vi "Global Log Handling Capability Example.vi"() -> ()   [LabVIEW 2017]
uses:
  user.lib/_NEVSTOP/Communicable State Machine(CSM)/Utility/_support/Periodic String Filter Level.ctl
  user.lib/_NEVSTOP/Communicable State Machine(CSM)/Utility/Periodic String Filter Setting.ctl
  user.lib/_NEVSTOP/Communicable State Machine(CSM)/Communicable State Machine.lvlib
  user.lib/_NEVSTOP/Communicable State Machine(CSM)/addons/Watchdog/CSM Watchdog.lvlib
  user.lib/_NEVSTOP/Communicable State Machine(CSM)/_Shared/CSM Shared.lvlib
panel:
  in  "Module Num":i32=30
  out "log handling Speed(#/s)":dbl(graph)
  out "Since Exiting(s)":dbl format="%.2f"
  out "LogInQ":i32
  out "State History":string
  out "log handling Speed(#/s)":dbl
  out "LogInQ changing Speed(#/s)":dbl
  out "Level":T1
  out "Module Names":string[](array[string])
  in  "Exit Modules":bool
  # "Set before run VI"
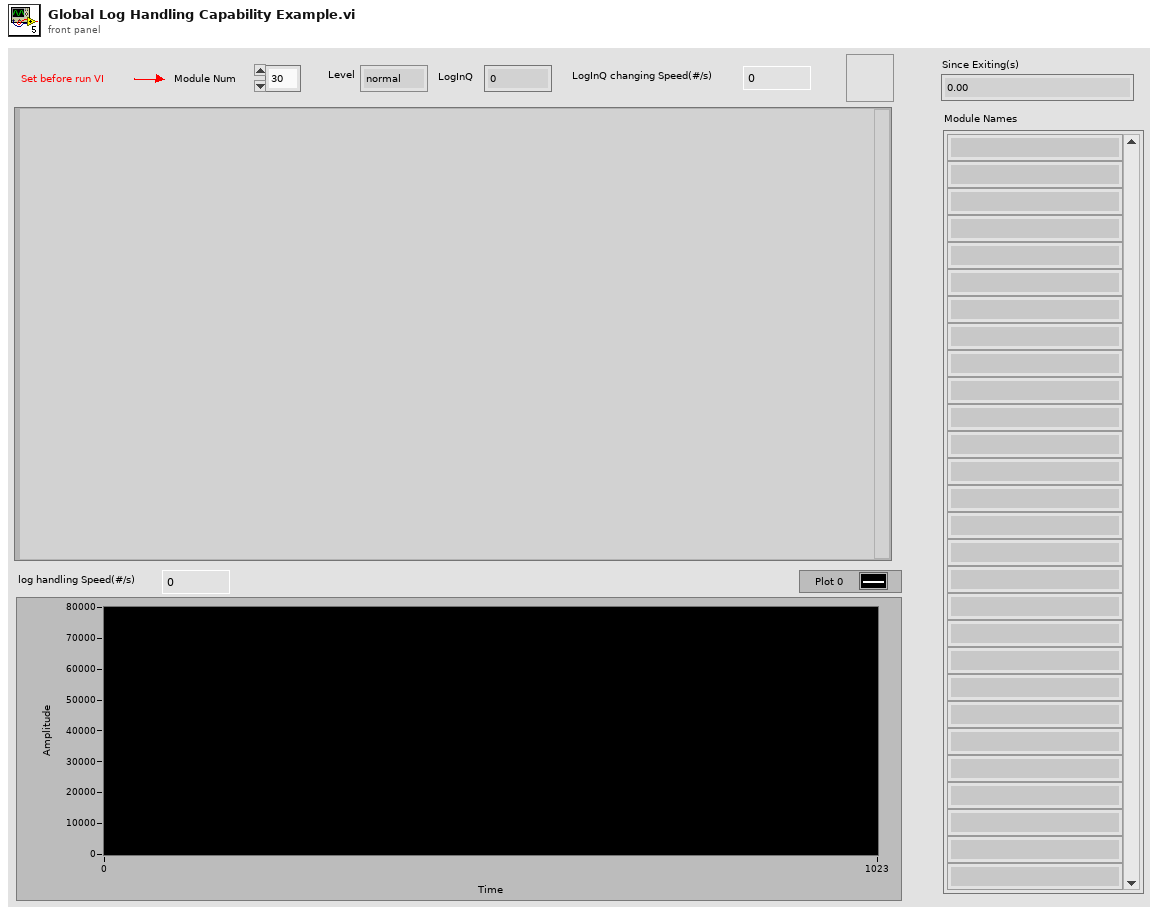
[diagram p1: front panel]
types:
  T1 = typedef "Communicable State Machine.lvlib/Periodic String Filter Level.ctl" = enum16{"normal", "L1", "L2", "L3", "L4"}
  T2 = typedef "Communicable State Machine.lvlib/Periodic String Filter Setting.ctl" = cluster{"threashold(#/s)":dbl, "Check Peroid(s)":dbl}
  T3 = typedef "Communicable State Machine.lvlib/_CSM_GlobalLog_MSG.ctl" = cluster{"Name(\"\" to use uuid)":string, "Current State":string, "Arguments":string, "Source Message":T4, "Source Module":string, "Complete(T)/Start(F)":bool, "LogType":T5, "Time Stamp":timestamp}
  T4 = typedef "Communicable State Machine.lvlib/_CSM_Response Source Message.ctl" = cluster{"‘State":string, "’Arguments":string, "’Error":errorcluster}
  T5 = typedef "Communicable State Machine.lvlib/_CSM_GlobalLog_MSG_TYPE.ctl" = enum16{"User Log", "State Change", "Status", "Interrupt", "Register", "Unregister", "Error Log", "Module Created", "Module Destroyed"}
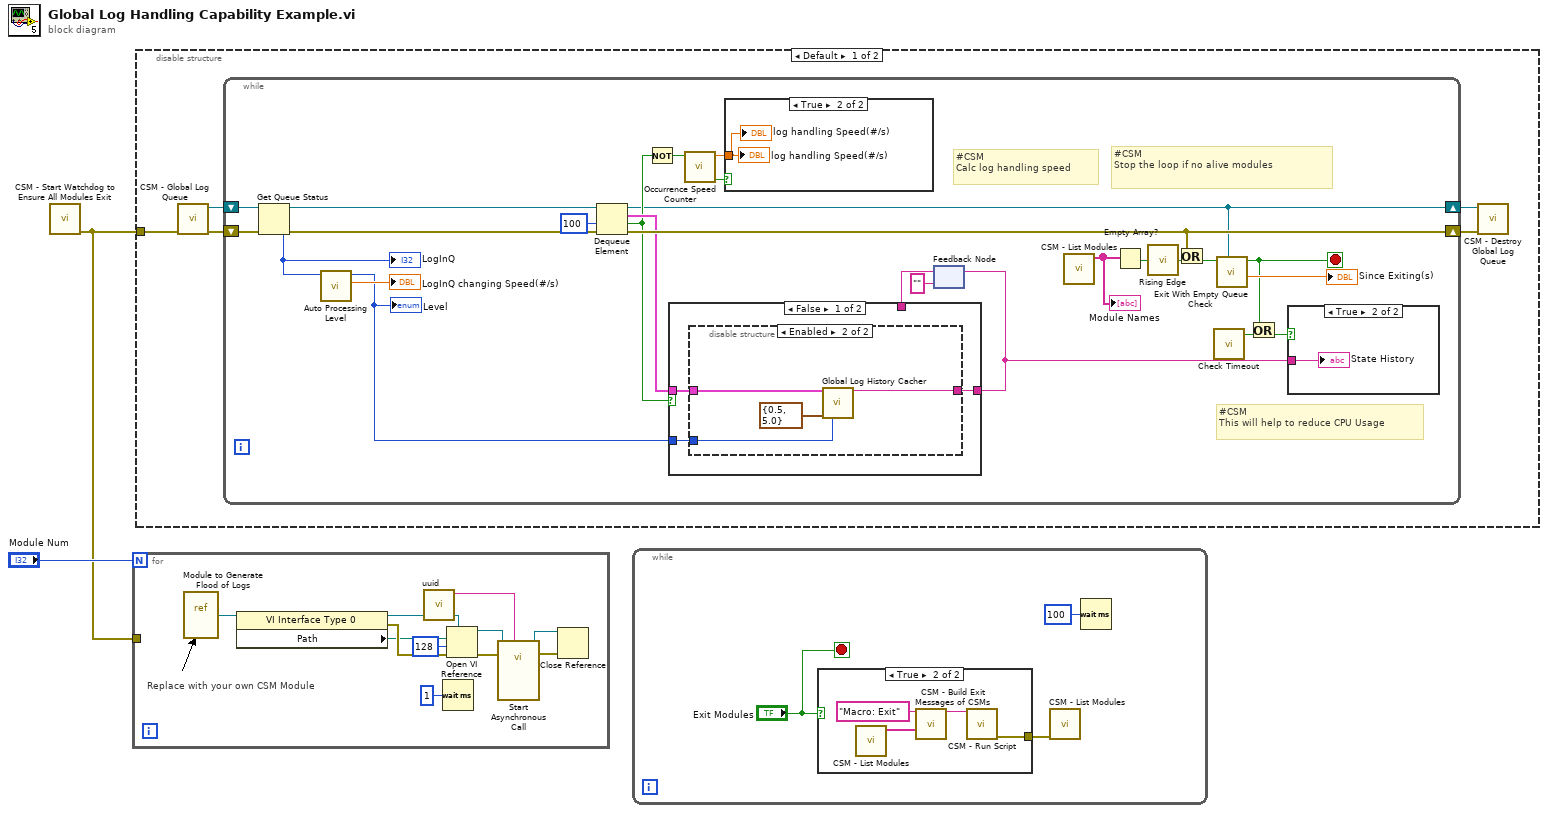
[diagram p0: block diagram]
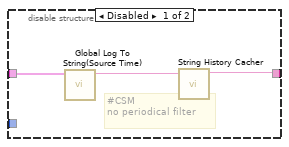
[diagram p3: hidden frame]
diagram:
  n1 = call "CSM - Start Watchdog to Ensure All Modules Exit.vi"() -> ("error out"=w1:errorcluster)  [unwired: 11 in]
  n2 = for {
    N: "Module Num" -> [_]
    tunnel: w1 -> [_]
    # "Replace with your own CSM Module"
    n3 = vi-ref "Module to Generate Flood of Logs.vi"() -> (w6:refnum<vi>)
    n4 = property class="VI Interface Type 0"(reference=w6) -> (reference out=w10:refnum<vi>, error out=w8:errorcluster, "Path"=w7:path)  [unwired: 1 in]
    n5 = call "uuid.vi"() -> ("UUID"=w4:string)  [unwired: 11 in]
    n6 = Wait (ms)(milliseconds to wait=u32 1) -> ()  [unwired: 1 out]
    n7 = Open VI Reference(type specifier VI Refnum (for type only)=w10, vi path=w7, options=128, error in (no error)=w8) -> (vi reference=w9:refnum<vi>, error out=w5:errorcluster)  [unwired: 2 in]
    n8 = call-by-ref "Start Asynchronous Call"(reference=w9, error in=w5, "Name(\"\" to use uuid)"=w4) -> (reference out=w12:refnum<vi>, error out=w11:errorcluster)  [unwired: 11 in]
    n9 = Close Reference(reference=w12, error in (no error)=w11) -> ()  [unwired: 1 out]
  }
  n10 = disable-structure shown="Default" {
    disable-tunnel: w1 -> [w14 _]
    frame condition #0 (active) {
      n11 = call "CSM - Global Log Queue.vi"("Error in"=w14) -> ("Error out"=w17:errorcluster, "GlobalEvent Queue"=w15:refnum<queue>)  [unwired: 9 in]
      n12 = while {
        shift-right: [w43] -> w18
        shift-left: w17 -> [w40]
        shift-right: [w31] -> w16
        shift-left: w15 -> [w44]
        stop <- w23 stop-if-true
        # "#CSM\nCalc log handling speed"
        # "#CSM\nStop the loop if no alive modules"
        # "#CSM\nThis will help to reduce CPU Usage"
        n13 = Get Queue Status(queue=w44, error in (no error)=w40) -> (queue out=w42:refnum<queue>, error out=w41:errorcluster, # elements in queue=w27:i32)  [unwired: 1 in, 5 out]
        "LogInQ" <- w27
        n14 = call "Auto Processing Level.vi"("#Left In Q"=w27) -> ("LogInQ changing Speed(#/s)"=→"LogInQ changing Speed(#/s)":dbl, "Level"=w26:T1)  [unwired: 8 in, 1 out]
        "Level" <- w26
        n15 = Dequeue Element(queue=w42, timeout in ms (-1)=100, error in (no error)=w41) -> (queue out=w31:refnum<queue>, element=w39:T3, timed out?=w33:bool, error out=w43:errorcluster)
        n16 = Not(x=w33) -> (.not. x?=w32:bool)
        n17 = call "Occurrence Speed Counter.vi"("Occured?(T)"=w32) -> ("New?"=w21:bool, "Speed(#/s)"=w22:dbl)  [unwired: 8 in, 1 out]
        n18 = case shown="True" w21 {
          tunnel: w22 -> [_ w45]
          frame False {
          }
          frame True {
            "log handling Speed(#/s)" <- w45
            "log handling Speed(#/s)" <- w45
          }
        }
        n19 = feedback #1("" ("String Cache")) -> (w35:string)
        n20 = case shown="False" w33 {
          tunnel: w39 -> [w48 _]
          tunnel: [w47 w56] -> w36
          tunnel: w35 -> [_ w56]
          tunnel: w26 -> [w46 _]
          frame False {
            n21 = disable-structure shown="Enabled" {
              disable-tunnel: w48 -> [w51 w54]
              disable-tunnel: [w49 w55] -> w47
              disable-tunnel: w46 -> [_ w53]
              frame Disabled {
                # "#CSM \nno periodical filter"
                n22 = call "Global Log To String(Source Time).vi"("Log"=w51) -> ("Log String"=w50:string)  [unwired: 9 in]
                n23 = call "String History Cacher.vi"("String"=w50) -> ("String Cache"=w49:string)  [unwired: 10 in]
              }
              frame Enabled {
                n24 = call "Global Log History Cacher.vi"("Cross CSM Data"=w54, "Settings"=T2 {"threashold(#/s)"=0.5, "Check Peroid(s)"=5.0}, "Level(Normal)"=w53) -> ("String Cache"=w55:string)  [unwired: 12 in]
              }
            }
          }
          frame True {
          }
        }
        n25 = feedback-in #1(w36) -> ()
        n26 = call "CSM - List Modules.vi"() -> ("Module Names"=w24:string[])  [unwired: 10 in, 1 out]
        "Module Names" <- w24
        n27 = Empty Array?(array=w24) -> (empty?=w20:bool)
        n28 = call "Rising Edge.vi"("signal"=w20) -> ("rising edge"=w19:bool)
        n29 = Or(x=w43, y=w19) -> (x .or. y?=w29:bool)
        n30 = call "Check Timeout.vi"() -> ("Timeout"=w37:bool)  [unwired: 8 in]
        n31 = call "Exit With Empty Queue Check.vi"("queue"=w31, "Stop"=w29) -> ("Since Exiting(s)"=→"Since Exiting(s)":dbl, "exit"=w23:bool)  [unwired: 8 in]
        n32 = Or(x=w23, y=w37) -> (x .or. y?=w30:bool)
        n33 = case shown="True" w30 {
          tunnel: w36 -> [_ w57]
          frame False {
          }
          frame True {
            "State History" <- w57
          }
        }
      }
      n34 = call "CSM - Destroy Global Log Queue.vi"("Error in"=w18, "CreatedQueue"=w16) -> ()  [unwired: 9 in, 1 out]
    }
    frame condition #1 {
    }
  }
  n35 = while {
    stop <- "Exit Modules" stop-if-true
    n36 = case shown="True" "Exit Modules" {
      tunnel: [_ w62] -> w59
      frame False {
      }
      frame True {
        n37 = call "CSM - List Modules.vi"() -> ("Module Names"=w64:string[])  [unwired: 10 in, 1 out]
        n38 = call "CSM - Build Exit Messages of CSMs.vi"("State with Arguments(\"Macro: Exit“)"="Macro: Exit" ("State with Arguments(\"Macro: Exit“)"), "CSMs"=w64) -> ("States"=w61:string)  [unwired: 13 in]
        n39 = call "CSM - Run Script.vi"("CSM Scripts"=w61) -> ("error out"=w62:errorcluster)  [unwired: 12 in, 2 out]
      }
    }
    n40 = call "CSM - List Modules.vi"("Error in"=w59) -> ()  [unwired: 9 in, 2 out]
    n41 = Wait (ms)(milliseconds to wait=u32 100) -> ()  [unwired: 1 out]
  }
